vi "Shooter Controller.vi"(8 "error in":errorcluster) -> ()   [LabVIEW 2016]
doc: "This VI executes continuously carrying out the current operation and responding to updates or new operations. It will often contain the timing or control code that is difficult to place directly in TeleOp. This VI generally opens all sensors and motors and isolates the rest of the robot code from knowing how the operations are carried out."
uses:
  Shooter Setpoints.ctl
  Shooter Operations.ctl
  <vilib>/Rock Robotics/WPI/ThirdParty/CanMotor/TalonSRX/WPI_CANTalonSRX_APIControlMode.ctl
  <vilib>/Rock Robotics/WPI/ThirdParty/CanMotor/TalonSRX/WPI_CANTalonSRX_APIFeedbackSelect.ctl
  <vilib>/Rock Robotics/Network Tables/NT Write Boolean.vi
panel:
  out "Current\nCmd":string
  # "Tip: It may be helpful to observe inputs and sensor values.\nYou may also want to display tuning or debugging controls."
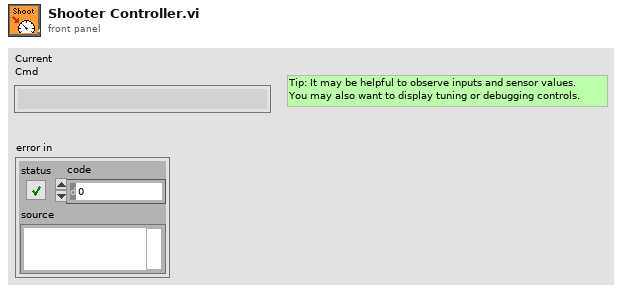
[diagram p1: front panel]
types:
  T1 = typedef "WPI_CANTalonSRX_APIFeedbackSelect.ctl" = enum16{"Digital Quadrature Encoder", "Analog Potentiometer", "Analog Encoder", "Count on Quad-A (Rising-Edge)", "Count on Quad-A (Falling-Edge)", "CTR Magnetic Enc (Absolute)", "CTR Magnetic Enc (Relative)", "Pulse Width"}
  T2 = typedef "WPI_CANTalonSRX_APIControlMode.ctl" = enum8{"Percent VBus", "Speed", "Position", "Slave", "Unchanged / Invalid", "Voltage Compensation", "Current", "Motion Profile", "Motion Magic"}
  T3 = typedef "Shooter Setpoints.ctl" = cluster{"Operation":T4, "Setpoint":dbl, "Duration":dbl}
  T4 = typedef "Shooter Operations.ctl" = enum16{"Reserve", "Read Current", "Immediate"}
  T5 = typedef "WPI_MotorControlDeviceRef.ctl" = cluster{"DeviceStatus":errorcluster, "Type":T6, "PWM":cluster{"PWM Channel":T7, "DeadBand":T8}, "CAN":cluster{"Device Number":u8, "SetOutput VI Ref":variant, "GetOutput VI Ref":variant, "Enable VI Ref":variant, "Disable VI Ref":variant, "Data":variant}, "Invert":bool}
  T6 = typedef "WPI_MotorControlType.ctl" = enum16{"PWM", "CAN"}
  T7 = typedef "FPGA_DIOPWMChannel.ctl" = enum8{"PWM 0", "PWM 1", "PWM 2", "PWM 3", "PWM 4", "PWM 5", "PWM 6", "PWM 7", "PWM 8", "PWM 9", "PWM MXP 0", "PWM MXP 1", "PWM MXP 2", "PWM MXP 3", "PWM MXP 4", "PWM MXP 5", "PWM MXP 6", "PWM MXP 7", "PWM MXP 8", "PWM MXP 9", "Invalid"}
  T8 = typedef "WPI_PWMDeadband.ctl" = cluster{"Name":string, "maxPositivePwm":i32, "minPositivePwm":i32, "centerPwm":i32, "maxNegativePwm":i32, "minNegativePwm":i32, "angularRange":u16}
  T9 = typedef "Command Status Info.ctl" = cluster{"Name":string, "Status":T10, "notifier out":T11}
  T10 = typedef "Completion Status.ctl" = enum16{"Successful", "Aborted", "Incomplete"}
  T11 = typedef "Completion Notifier.ctl" = refnum<notifier>
  T12 = cluster{"Default Command":T3, "Command Timing":cluster{"Start Time (ms)":u32, "Iterations":i32}, "Command Arguments":cluster{"Command Info":T9, "Description":string, "Default Command":T3, "notifier out":refnum<notifier>, "Subsystem Name":string}}
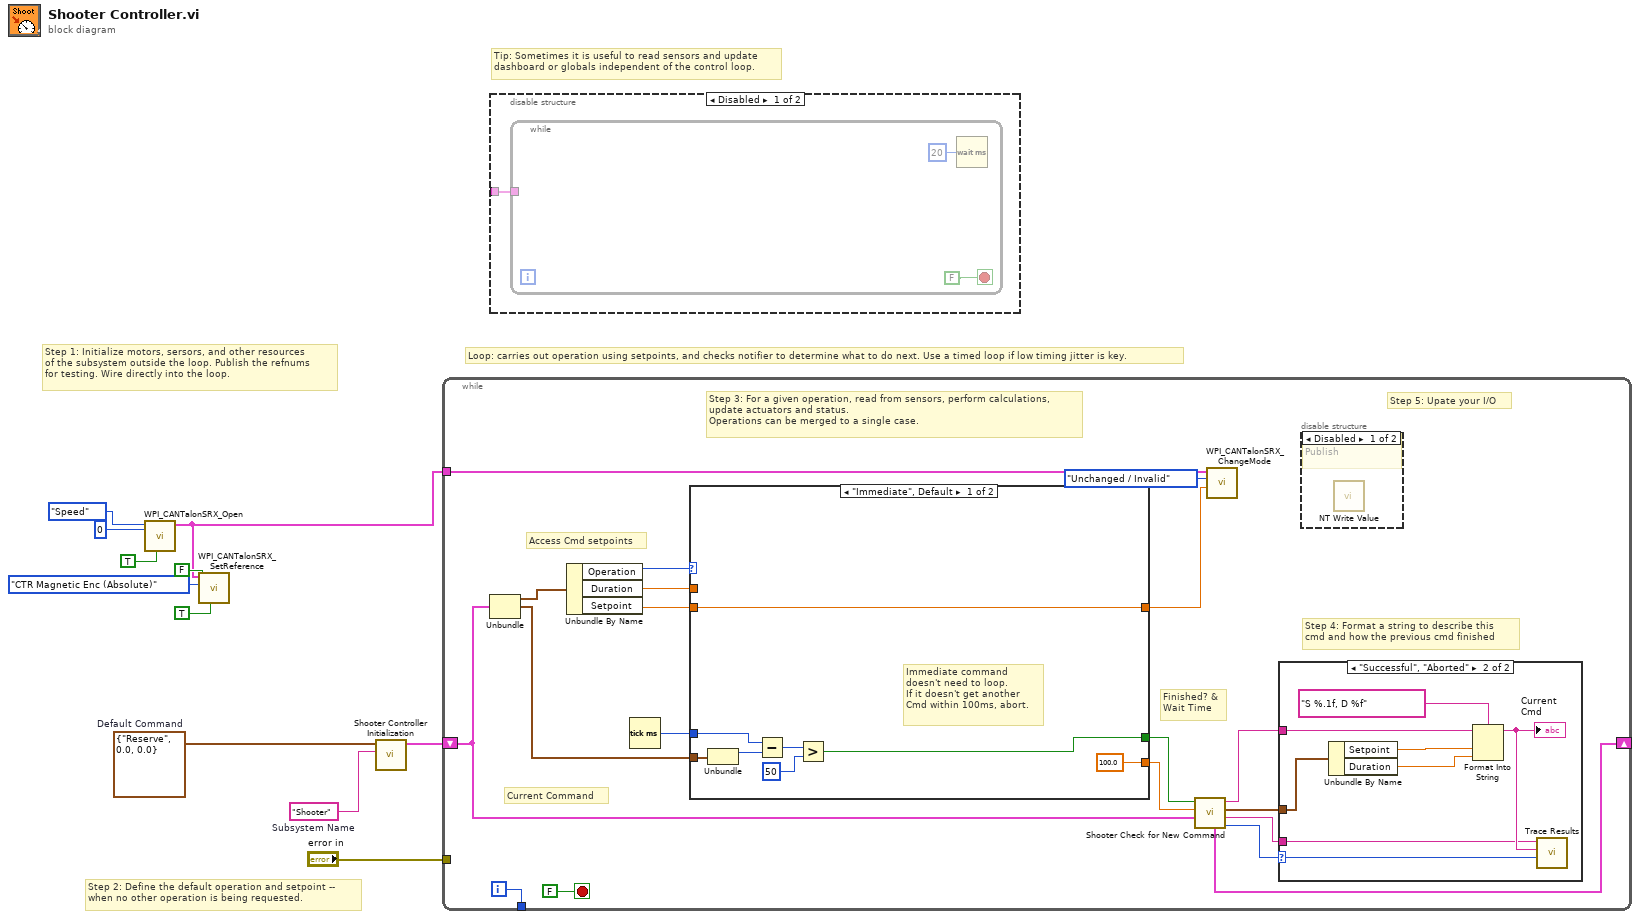
[diagram p0: block diagram]
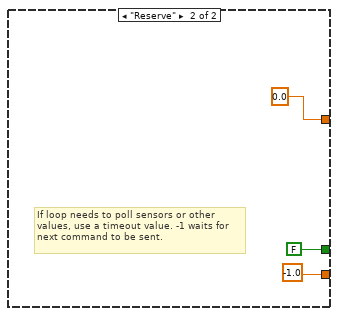
[diagram p5: hidden frame]
diagram:
  w8 = T3 {"Operation"=enum."Reserve", "Setpoint"=0.0, "Duration"=0.0}  # Default Command
  w9 = "Shooter"  # Subsystem Name
  # "Tip: Sometimes it is useful to read sensors and update\ndashboard or globals independent of the control loop."
  # "Step 2: Define the default operation and setpoint --\nwhen no other operation is being requested."
  # "Step 1: Initialize motors, sersors, and other resources\nof the subsystem outside the loop. Publish the refnums\nfor testing. Wire directly into the loop."
  # "Loop: carries out operation using setpoints, and checks notifier to determine what to do next. Use a timed loop if low timing jitter is key."
  n1 = call <vilib>:"WPI_CANTalonSRX_Open.vi"("Invert"=TRUE, "Device Number"=u8 0, "Control Mode"=WPI_CANTalonSRX_APIControlMode."Speed") -> ("CAN Talon SRX Ref"=w1:T5)  [unwired: 7 in, 1 out]
  n2 = call <vilib>:"WPI_CANTalonSRX_SetReference.vi"("Reverse Closed-Loop Output"=TRUE, "Reverse Feedback Sensor"=FALSE, "Feedback Reference"=WPI_CANTalonSRX_APIFeedbackSelect."CTR Magnetic Enc (Absolute)", "CAN Talon SRX Ref"=w1) -> ()  [unwired: 6 in, 2 out]
  n3 = call "Shooter Controller Initialization.vi"("Subsystem Name"=w9, "Default Command"=w8) -> ("Command Info"=w10:T12)  [unwired: 9 in]
  n4 = while {
    shift-right: [w21] -> _
    shift-left: w10 -> [w22]
    tunnel: [w29] -> _
    tunnel: "error in" -> [_]
    tunnel: w1 -> [w14]
    i -> [w29]
    stop <- FALSE stop-if-true
    # "Step 5: Upate your I/O"
    # "Step 4: Format a string to describe this\ncmd and how the previous cmd finished"
    # "Current Command"
    # "Access Cmd setpoints"
    # "Finished? &\nWait Time"
    # "Step 3: For a given operation, read from sensors, perform calculations,\nupdate actuators and status.\nOperations can be merged to a single case."
    n5 = Unbundle(w22) -> ("Default Command"=w28:T3, "Command Timing"=w24:cluster{"Start Time (ms)":u32, "Iterations":i32})  [unwired: 1 out]
    n6 = Unbundle By Name(w28) -> ("Operation"=w27:T4, "Duration"=w26:dbl, "Setpoint"=w23:dbl)
    n7 = Tick Count (ms)() -> (millisecond timer value=w25:u32)
    n8 = case shown="\"Immediate\", Default" w27 {
      tunnel: [100.0 -1.0] -> w19
      tunnel: [w40 FALSE ("ignore previous (F)")] -> w20
      tunnel: w24 -> [w42 _]
      tunnel: w26 -> [_ _]
      tunnel: w25 -> [w41 _]
      tunnel: w23 -> [w39 _]
      tunnel: [w39 0.0] -> w12
      frame "Immediate", Default {
        # "Immediate command\ndoesn't need to loop.\nIf it doesn't get another\nCmd within 100ms, abort."
        n9 = Unbundle(w42) -> ("Start Time (ms)"=w45:u32)  [unwired: 1 out]
        n10 = Subtract(x=w41, y=w45) -> (x-y=w44:u32)
        n11 = Greater?(x=w44, y=u8 50 ("Left Motor")) -> (0:w40:bool)
      }
      frame "Reserve" {
        # "If loop needs to poll sensors or other\nvalues, use a timeout value. -1 waits for\nnext command to be sent."
      }
    }
    n12 = call "Shooter Check for New Command.vi"("Current Command"=w22, "Wait time (ms)"=w19, "Finished?"=w20) -> ("Completion"=w15:T10, "Subsystem Name"=w16:string, "Current Command"=w17:T3, "Initial Trace String"=w18:string, "NextCommand"=w21:T12)  [unwired: 4 in]
    n13 = call <vilib>:"WPI_CANTalonSRX_ChangeMode.vi"("Output"=w12, "Control Mode"=WPI_CANTalonSRX_APIControlMode."Unchanged / Invalid", "CAN Talon SRX Ref"=w14) -> ()  [unwired: 7 in, 2 out]
    n14 = case shown="\"Successful\", \"Aborted\"" w15 {
      selector: w15 -> [_ w38]
      tunnel: w18 -> [_ w34]
      tunnel: w17 -> [_ w35]
      tunnel: w16 -> [_ w31]
      frame "Incomplete", Default {
        # "Continuing current command"
      }
      frame "Successful", "Aborted" {
        # "Report and setup for next command"
        n15 = Unbundle By Name(w35) -> ("Setpoint"=w37:dbl, "Duration"=w32:dbl)
        n16 = Format Into String(format string="S %.1f, D %f", initial string=w34, w37, w32) -> (resulting string=w33:string)  [unwired: 1 in, 1 out]
        "Current\nCmd" <- w33
        n17 = call <vilib>:"Trace Results.vi"("Status of previous command"=w38, "Description"=w33, "Subsystem"=w31) -> ()  [unwired: 9 in]
      }
    }
    n18 = disable-structure shown="Disabled" {
      frame Disabled {
        # "Publish"
        n19 = call-poly <vilib>:"NT Write Value.vi"() -> ()  [unwired: 11 in, 1 out]
      }
      frame Enabled {
      }
    }
  }
  n20 = disable-structure shown="Disabled" {
    disable-tunnel: _ -> [w50 _]
    frame Disabled {
      n21 = while {
        tunnel: w50 -> [_]
        stop <- FALSE stop-if-true
        n22 = Wait (ms)(milliseconds to wait=u32 20) -> ()  [unwired: 1 out]
      }
    }
    frame Enabled {
    }
  }
